vi "SaveImageAtWell.vi"(7 "namespace":string, 8 "error in (no error)":errorcluster, 9 "Well":cluster{"X":u32, "Y":u32}, 10 "image data":T1, 11 "Microscope":refnum<class "Microscope.lvclass">) -> (0 "error out":errorcluster, 2 "image path":path, 3 "Microscope out":refnum<class "Microscope.lvclass">)   [LabVIEW 2015, in "Microscope.lvclass"]
doc: "---------------------------------------------------------------\nJKI State Machine Objects™\nhttp://jki.net/state-machine-objects/\nCopyright (C) 2005-2015, JKI <info@jki.net>\nALL RIGHTS RESERVEDJKI State Machine Objects (SMO) 1.0.0.4\nJKI - JKI\nCopyright (c) 2015, JKI"
uses:
  Microscope.lvclass
  <vilib>/picture/picture.llb/imagedata.ctl
  <userlib>/_OpenG.lib/file/file.llb/Build Path - Traditional__ogtk.vi
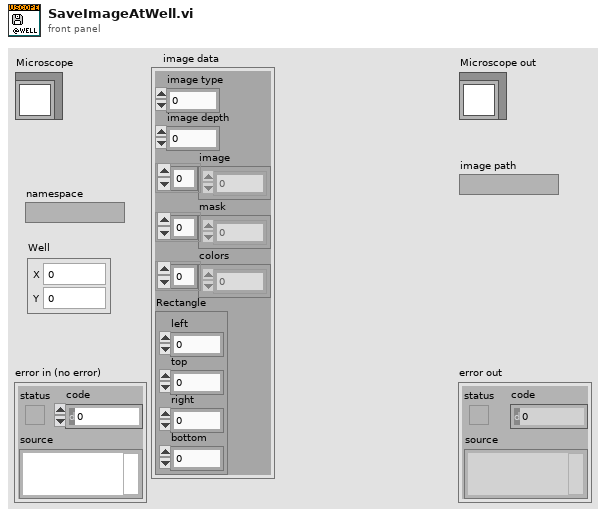
[diagram p1: front panel]
types:
  T1 = typedef "imagedata.ctl" = cluster{"image type":i32, "image depth":i32, "image":u8[], "mask":u8[], "colors":u32[], "Rectangle":cluster{"left":i16, "top":i16, "right":i16, "bottom":i16}}
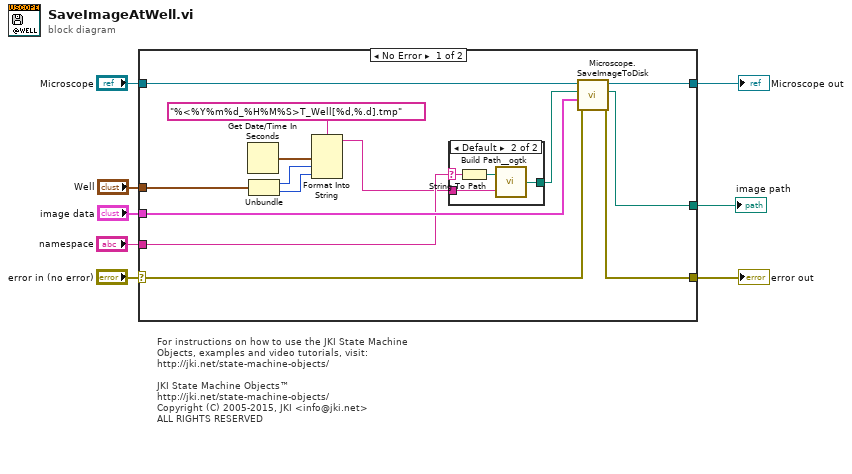
[diagram p0: block diagram]
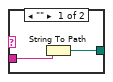
[diagram p2: hidden frame]
diagram:
  # "For instructions on how to use the JKI State Machine Objects, examples and video tutorials, visit:\nhttp://jki.net/state-machine-objects/\n\nJKI State Machine Objects™\nhttp://jki.net/state-machine-objects/\nCopyright (C) 2005-2015, JKI <info@jki.net>\nALL RIGHTS RESERVED"
  n1 = case shown="No Error" "error in (no error)" {
    selector: "error in (no error)" -> [w13 w30]
    tunnel: [w18 w30] -> w7
    tunnel: [w14 w29] -> w8
    tunnel: "Microscope" -> [w22 w29]
    tunnel: "image data" -> [w19 _]
    tunnel: "Well" -> [w21 _]
    tunnel: "namespace" -> [w12 _]
    tunnel: [w9 _] -> w1
    frame No Error {
      n2 = Get Date/Time In Seconds() -> (seconds since 1Jan1904=w17:timestamp)
      n3 = Unbundle(w21) -> ("X"=w16:u32, "Y"=w15:u32)
      n4 = Format Into String(format string="%<%Y%m%d_%H%M%S>T_Well[%d,%.d].tmp", w17, w16, w15) -> (resulting string=w11:string)  [unwired: 2 in, 1 out]
      n5 = case shown="Default" w12 {
        selector: w12 -> [_ w27]
        tunnel: [w24 w26] -> w10
        tunnel: w11 -> [w23 w28]
        frame "" {
          n6 = String To Path(string=w23) -> (path=w24:path)
        }
        frame Default {
          n7 = String To Path(string=w27) -> (path=w25:path)
          n8 = call-poly <userlib>:"Build Path__ogtk.vi"("name or relative path"=w28, "base path"=w25) -> ("appended path"=w26:path)
        }
      }
      n9 = call "Microscope.SaveImageToDisk.vi"("error in (no error)"=w13, "image data"=w19, "folder"=w10, "Microscope in"=w22) -> ("error out"=w18:errorcluster, "path out"=w9:path, "Microscope out"=w14:refnum<class "Microscope.lvclass">)  [unwired: 5 in]
    }
    frame Error {
    }
  }
  "error out" <- w7
  "Microscope out" <- w8
  "image path" <- w1
